vi "Joints to Angle XY.vi"(9 "Mirror":bool, 10 "Origin Joint":cluster{"x":sgl, "y":sgl, "z":sgl}, 11 "Moving Joint":cluster{"x":sgl, "y":sgl, "z":sgl}) -> (0 "In-Plane":bool, 3 "Angle":dbl)   [LabVIEW 2012]
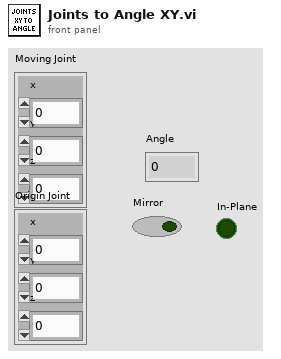
[diagram p1: front panel]
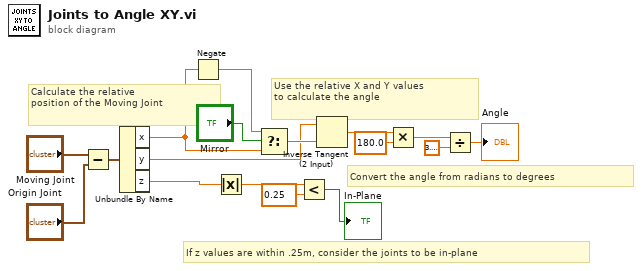
[diagram p0: block diagram]
diagram:
  # "Convert the angle from radians to degrees"
  # "Use the relative X and Y values\nto calculate the angle"
  # "Calculate the relative\nposition of the Moving Joint"
  # "If z values are within .25m, consider the joints to be in-plane"
  n1 = Subtract(x="Moving Joint", y="Origin Joint") -> (x-y=w12:cluster{"x":sgl, "y":sgl, "z":sgl})
  n2 = Unbundle By Name(w12) -> ("x"=w11:sgl, "y"=w7:sgl, "z"=w6:sgl)
  n3 = Negate(x=w11) -> (-x=w8:sgl)
  n4 = Absolute Value(x=w6) -> (abs(x)=w5:sgl)
  n5 = Select(t=w8, s="Mirror", f=w11) -> (s? t:f=w9:sgl)
  n6 = Less?(x=w5, y=sgl 0.25) -> (x < y?=→"In-Plane":bool)
  n7 = Inverse Tangent (2 Input)(1:w9, 2:w7) -> (0:w13:sgl)
  n8 = Multiply(x=w13, y=sgl 180.0) -> (x*y=w15:sgl)
  n9 = Divide(x=w15, y=3.141592653589793) -> (x/y=→"Angle":dbl)
